vi "BuildCustomDashBoardData.vi"() -> ()   [LabVIEW 2013]
doc: "This VI builds data and sends it back to the dashboard PC program. By default it sends back the raw values for the first analog, digital, and solenoid module. Modify it to send back the data you want to view. Consider adding higher level data to the Dashboard Datatype.ctl and to this VI. Then update the Dashboard to display the data however you like.\n\nThis software is licensed. Open the labview\\readme\\WPI Robotics Library Open Source License.txt file for more information."
uses:
  typedefs/Dashboard/DashboardEnable.ctl
  typedefs/fg_typedef.ctl
  <vilib>/Rock Robotics/SystemInterfaces/Typedef/FPGA_TypedefDigitalModule.ctl
  typedefs/Dashboard/dash dio.ctl
  typedefs/Dashboard/misc dash data.ctl
  typedefs/Dashboard/dashboard safety status data.ctl
  typedefs/Dashboard/dash error type def.ctl
  <vilib>/Rock Robotics/SystemInterfaces/System/FPGA_SystemGet.vi
  <vilib>/NI_Real-Time Target Support.lvlib
  <vilib>/Rock Robotics/WPI/DriverStation/WPI_DriverStationDigitalData.ctl
  typedefs/State Machine/subStates.ctl
  typedefs/Dashboard/custom dash data.ctl
  typedefs/Dashboard/Dashboard Datatype.ctl
panel:
  out "Errors":errorcluster
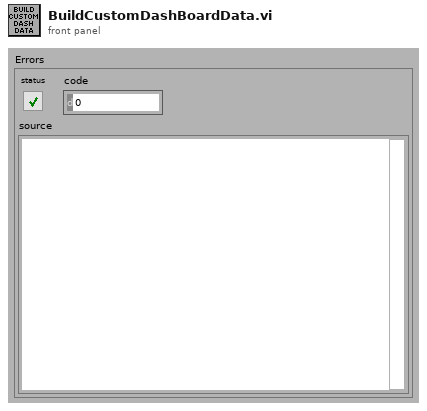
[diagram p1: front panel]
types:
  T1 = typedef "Dashboard Datatype.ctl" = cluster{cluster{"AnalogModule[0]":cluster{"Channel[0]":sgl, "Channel[1]":sgl, "Channel[2]":sgl, "Channel[3]":sgl, "Channel[4]":sgl, "Channel[5]":sgl, "Channel[6]":sgl, "Channel[7]":sgl}, "AnalogModule[1]":cluster{"Channel[0]":sgl, "Channel[1]":sgl, "Channel[2]":sgl, "Channel[3]":sgl, "Channel[4]":sgl, "Channel[5]":sgl, "Channel[6]":sgl, "Channel[7]":sgl}}, cluster{"DigitalModule[0]":T2, "DigitalModule[1]":T2}, "Solenoid":u8}
  T2 = typedef "WPI_DriverStationDigitalData.ctl" = cluster{"Relay Fwd":u8, "Relay Rev":u8, "GPIO":u16, "GPIO_OE":u16, "PWM":cluster{"PWM[0]":u8, "PWM[1]":u8, "PWM[2]":u8, "PWM[3]":u8, "PWM[4]":u8, "PWM[5]":u8, "PWM[6]":u8, "PWM[7]":u8, "PWM[8]":u8, "PWM[9]":u8}}
  T3 = typedef "custom dash data.ctl" = cluster{"Motors":cluster{"Pickup Motor":dbl, "Pickup Belt":dbl, "Pickup Distance ":dbl, "Pickup Rate":dbl, "Right Motor Rate":dbl, "Left Motor Rate":dbl, "Right Motor Distance":dbl, "Left Motor Distance":dbl}, "substates":cluster{"Latch":T4, "Pickup Arm":T4, "Belts":T4, "Shooter":T4, "Drive":T4}, "Safeties":cluster{"Arm Safety":bool, "Arm Limit":bool}, "Performance":cluster{"CPU Usage":dbl, "Vision mSPI":u32, "Main mSPI":u32}, "Vision Enabled?":bool, "Can Shoot Safely?":bool, "Timeout Error":cluster{"# of Timeouts":u32, "Time Out Error This Match":bool}, "Error FG Data":cluster{"Errors Present":bool, "Errors":string}, "Vision Data":cluster{"Hot Goal Present?":bool, "distance":dbl}}
  T4 = typedef "subStates.ctl" = enum16{"null", "wait", "driver control", "auto", "manual override", "hold position", "rotate", "pickup", "pass", "recover pass", "load", "goto shoot", "shoot high goal", "shoot low goal", "cancel arm", "cancel shooter", "end", "test"}
  T5 = typedef "fg_typedef.ctl" = enum16{"Get", "Set"}
  T6 = cluster{"# of Timeouts":u32, "Time Out Error This Match":bool}
  T7 = typedef "FPGA_TypedefDigitalModule.ctl" = enum16{"Digital Module 1", "Digital Module 2"}
  T8 = typedef "dash dio.ctl" = cluster{"Relay Forward":u8, "Relay Reverse":u8, u32, u32, cluster{"[0]":u8, "[1]":u8, "[2]":u8, "[3]":u8, "[4]":u8, "[5]":u8, "[6]":u8, "[7]":u8, "[8]":u8, "[9]":u8}}[]
  T9 = typedef "misc dash data.ctl" = cluster{"Total (%)":dbl, "Vision mSPI":u32, "Main mSPI":u32, "Vision":cluster{"Hot Goal Present?":bool, "distance":dbl}, "Enabled?":bool, "Safety Data":T10}
  T10 = typedef "dashboard safety status data.ctl" = cluster{"At Distance Limit":bool, "No Rate Read":bool, "Encoder Disconnected":bool, "Encoder Directional Issue":bool}
  T11 = typedef "dash error type def.ctl" = cluster{"Timeout Data":cluster{"# of Timeouts":u32, "Time Out Error This Match":bool}, "Can Shoot Safely?":bool}
  T12 = typedef "DashboardEnable.ctl" = cluster{"Analog Module 1":bool[], "Analog Module 2":bool[], "Digital Module 1":bool, "Digital Module 2":bool, "Solenoid Module":bool}
  T13 = cluster{"AnalogModule[0]":cluster{"Channel[0]":sgl, "Channel[1]":sgl, "Channel[2]":sgl, "Channel[3]":sgl, "Channel[4]":sgl, "Channel[5]":sgl, "Channel[6]":sgl, "Channel[7]":sgl}, "AnalogModule[1]":cluster{"Channel[0]":sgl, "Channel[1]":sgl, "Channel[2]":sgl, "Channel[3]":sgl, "Channel[4]":sgl, "Channel[5]":sgl, "Channel[6]":sgl, "Channel[7]":sgl}}
  T14 = cluster{"DigitalModule[0]":T2, "DigitalModule[1]":T2}
  T15 = typedef "vision data.ctl" = cluster{"x":dbl, "y":dbl, "area":dbl, "width":dbl, "height":dbl, "Hot Goal Present?":bool, "distance":dbl}
  T16 = cluster{"Channel[0]":sgl, "Channel[1]":sgl, "Channel[2]":sgl, "Channel[3]":sgl, "Channel[4]":sgl, "Channel[5]":sgl, "Channel[6]":sgl, "Channel[7]":sgl}[]
  T17 = cluster{"Channel[0]":sgl, "Channel[1]":sgl, "Channel[2]":sgl, "Channel[3]":sgl, "Channel[4]":sgl, "Channel[5]":sgl, "Channel[6]":sgl, "Channel[7]":sgl}
  T18 = cluster{"AnalogModule[0][0]":sgl, "AnalogModule[0][1]":sgl, "AnalogModule[0][2]":sgl, "AnalogModule[0][3]":sgl, "AnalogModule[0][4]":sgl, "AnalogModule[0][5]":sgl, "AnalogModule[0][6]":sgl, "AnalogModule[0][7]":sgl}
  T19 = cluster{"[0]":cluster{"Channel[0]":sgl, "Channel[1]":sgl, "Channel[2]":sgl, "Channel[3]":sgl, "Channel[4]":sgl, "Channel[5]":sgl, "Channel[6]":sgl, "Channel[7]":sgl}, "[1]":cluster{"Channel[0]":sgl, "Channel[1]":sgl, "Channel[2]":sgl, "Channel[3]":sgl, "Channel[4]":sgl, "Channel[5]":sgl, "Channel[6]":sgl, "Channel[7]":sgl}}
  T20 = typedef "FPGA_DIODevRef.ctl" = cluster{"DevStatus":errorcluster, "Module":T7}
  T21 = cluster{"[0]":u8, "[1]":u8, "[2]":u8, "[3]":u8, "[4]":u8, "[5]":u8, "[6]":u8, "[7]":u8, "[8]":u8, "[9]":u8}
  T22 = typedef "FPGA_SolenoidDevRef.ctl" = cluster{"DevStatus":errorcluster, "Module":T23}
  T23 = typedef "FPGA_TypedefSolenoidModule.ctl" = enum16{"Solenoid Module 1", "Solenoid Module 2"}
  T24 = cluster{"Pickup Motor":dbl, "Pickup Belt":dbl, "Pickup Distance ":dbl, "Pickup Rate":dbl, "Right Motor Rate":dbl, "Left Motor Rate":dbl, "Right Motor Distance":dbl, "Left Motor Distance":dbl}
  T25 = cluster{"CPU Usage":dbl, "Vision mSPI":u32, "Main mSPI":u32}
  T26 = cluster{"Hot Goal Present?":bool, "distance":dbl}
  T27 = typedef "WPI_EncoderDevRef.ctl" = cluster{"DevStatus":errorcluster, "EncoderIndex":T28, "CounterIndex":T29, "DistancePerCount":dbl, "Decoding Type":T30}
  T28 = typedef "FPGA_EncoderIdx.ctl" = enum8{"Enc 0", "Enc 1", "Enc 2", "Enc 3", "Invalid"}
  T29 = typedef "FPGA_CounterCtrSystemIndex.ctl" = enum8{"Ctr 0", "Ctr 1", "Ctr 2", "Ctr 3", "Ctr 4", "Ctr 5", "Ctr 6", "Ctr 7", "Invalid"}
  T30 = typedef "WPI_EncoderType.ctl" = enum16{"1x", "2x", "4x"}
  T31 = typedef "WPI_MotorControlDeviceRef.ctl" = cluster{"DeviceStatus":errorcluster, "Type":enum16{"PWM", "CAN"}, "PWM":cluster{"Digital Module":T7, "PWM Channel":T32, "DeadBand":T33}, "CAN":cluster{"Device Number":u8, "Control Mode":T34, "Semaphore":T35, "Max Vout":dbl}, "Invert":bool, "TransformRef":T36, "InvTransformRef":T36}
  T32 = typedef "FPGA_DIOPWMChannel.ctl" = enum8{"PWM 1", "PWM 2", "PWM 3", "PWM 4", "PWM 5", "PWM 6", "PWM 7", "PWM 8", "PWM 9", "PWM 10", "Invalid"}
  T33 = typedef "WPI_PWMDeadband.ctl" = cluster{"Name":string, "maxPositivePwm":i32, "minPositivePwm":i32, "centerPwm":i32, "maxNegativePwm":i32, "minNegativePwm":i32, "angularRange":u16}
  T34 = typedef "WPI_CANJaguar_ControlMode.ctl" = enum8{"Percent VBus", "Current", "Speed", "Position", "Voltage"}
  T35 = typedef "Semaphore RefNum" = refnum<k1>
  T36 = typedef "WPI_PWMTransform_ConPane.ctl" = refnum<vi>
  T37 = typedef "NI_Real-Time Target Support.lvlib/RT CPU Load.ctl" = cluster{"Total (%)":dbl, "Time Critical (%)":dbl, "Timed Structures (%)":dbl, "High (%)":dbl, "Above Normal (%)":dbl, "Normal (%)":dbl, "Background (%)":dbl, "Idle (%)":dbl, "ISR (%)":dbl}
  T38 = cluster{"Vision mSPI":u32, "Main mSPI":u32, "Dash mSPI":u32}
  T39 = cluster{"Relay Forward":u8, "Relay Reverse":u8, u32, u32, cluster{"[0]":u8, "[1]":u8, "[2]":u8, "[3]":u8, "[4]":u8, "[5]":u8, "[6]":u8, "[7]":u8, "[8]":u8, "[9]":u8}}
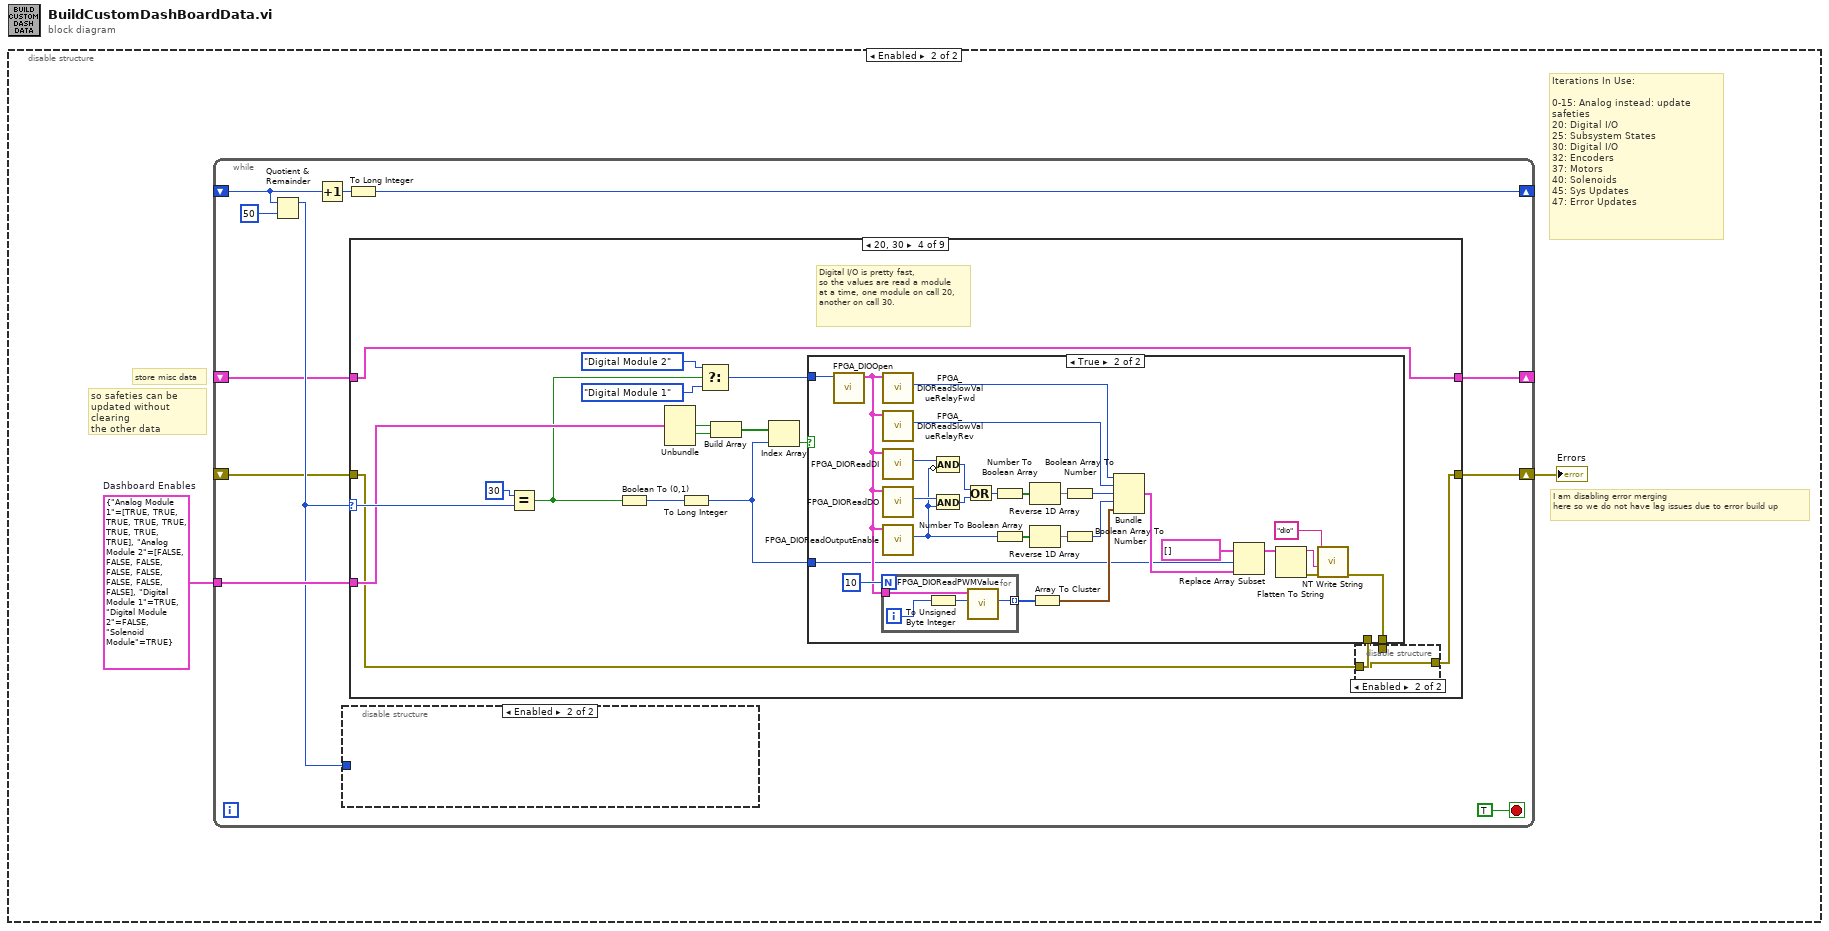
[diagram p0: block diagram]
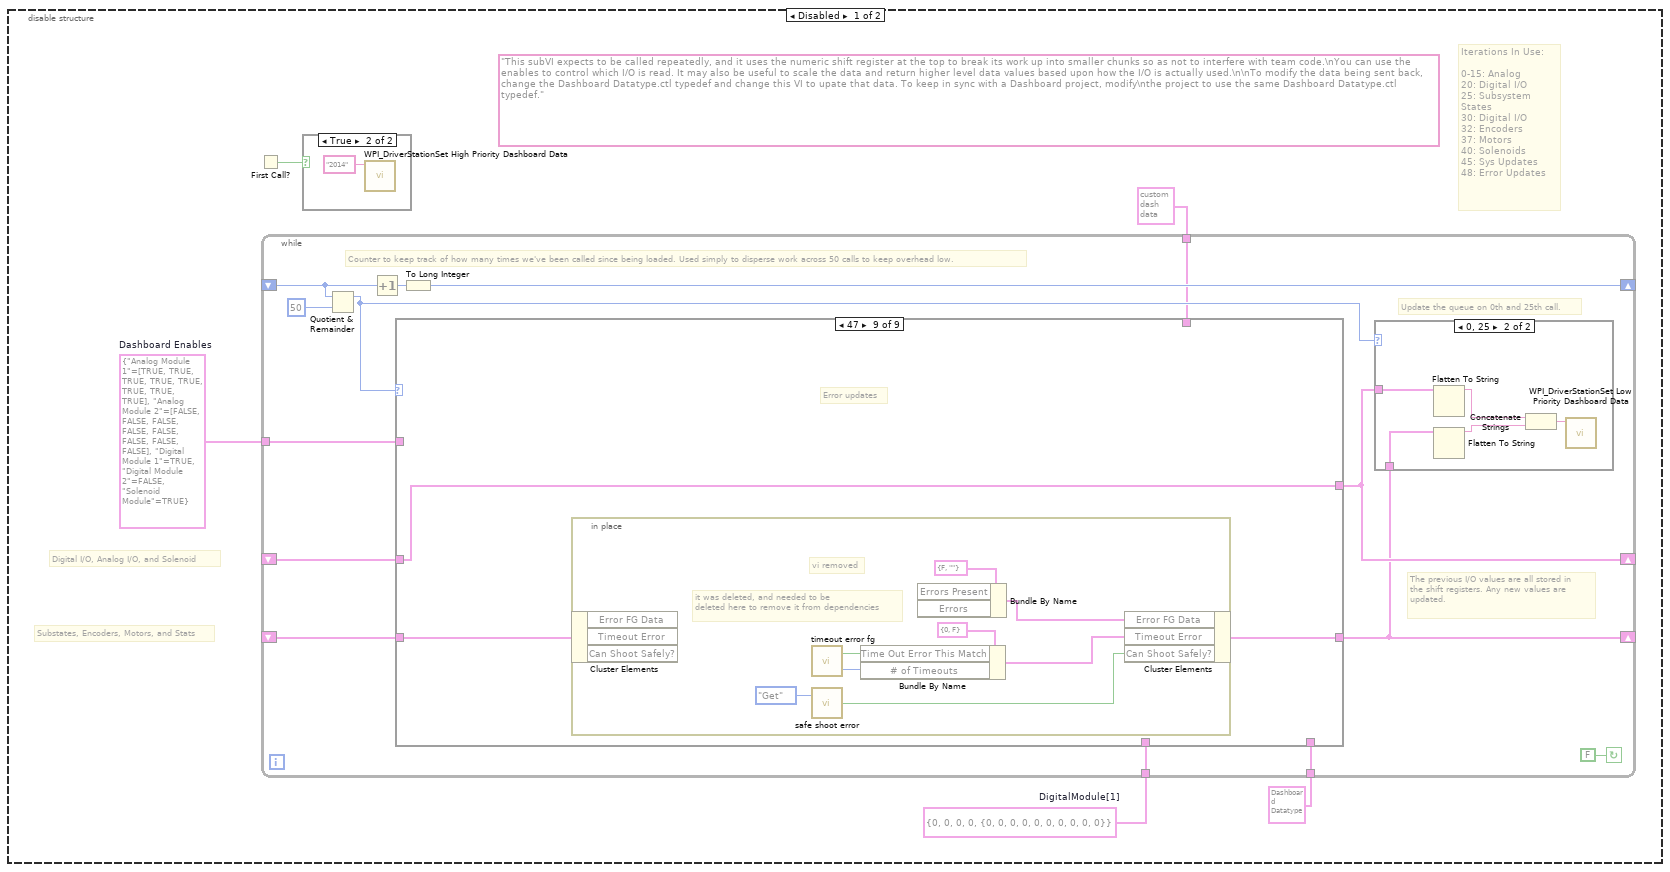
[diagram p2: hidden frame]
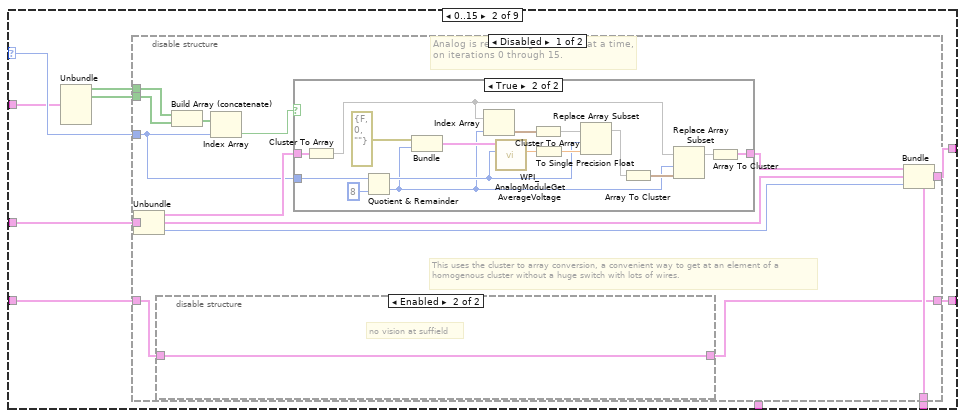
[diagram p6: hidden frame]
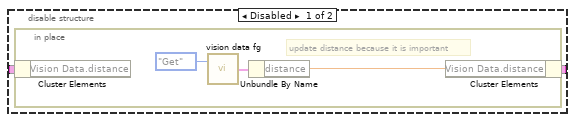
[diagram p8: hidden frame]
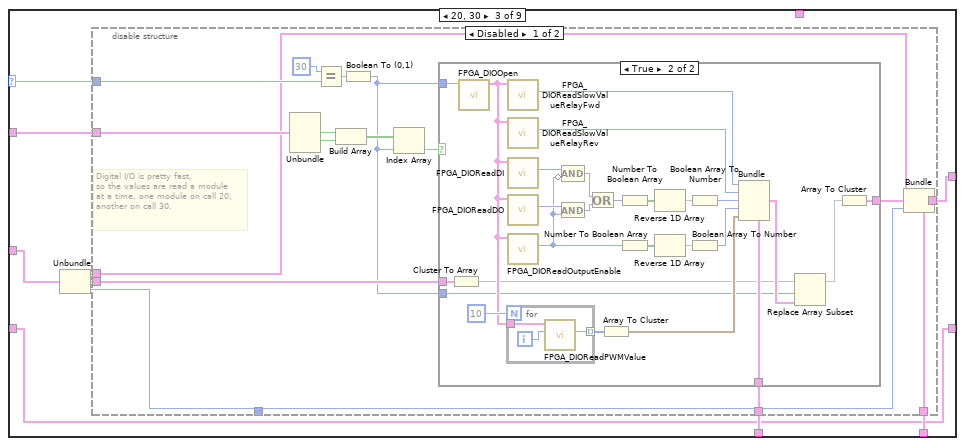
[diagram p10: hidden frame]
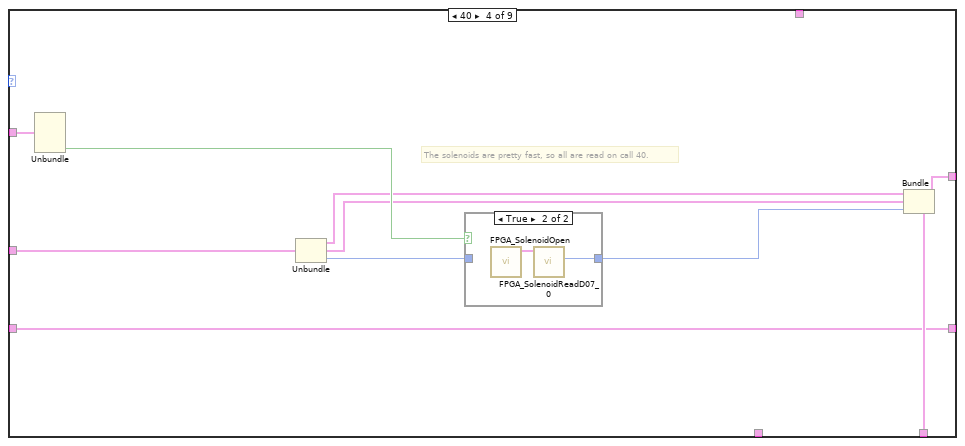
[diagram p13: hidden frame]
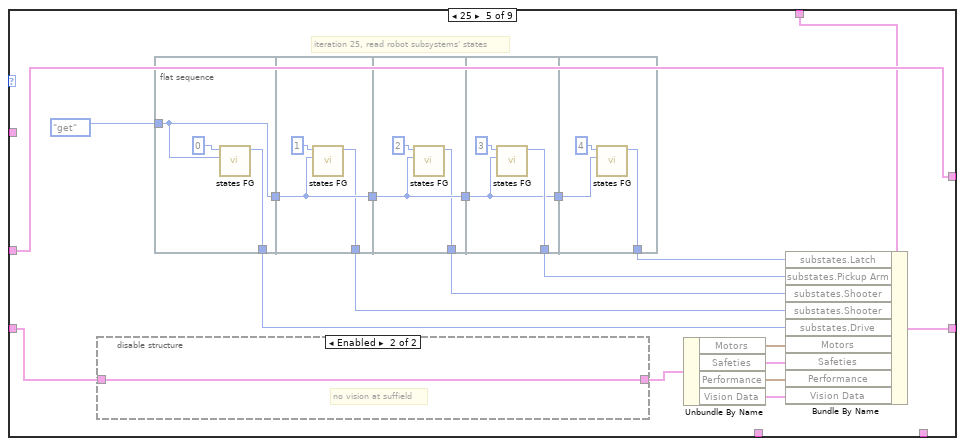
[diagram p15: hidden frame]
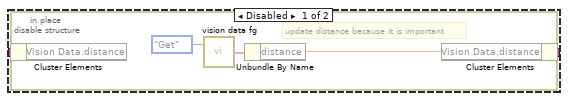
[diagram p16: hidden frame]
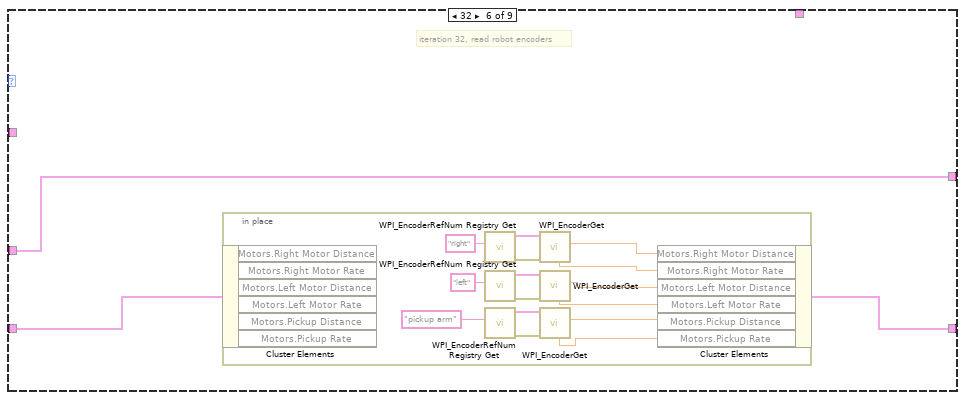
[diagram p17: hidden frame]
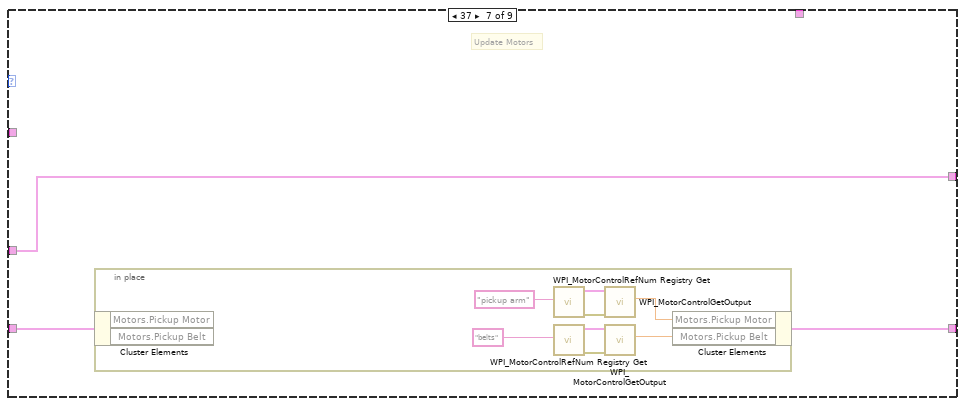
[diagram p18: hidden frame]
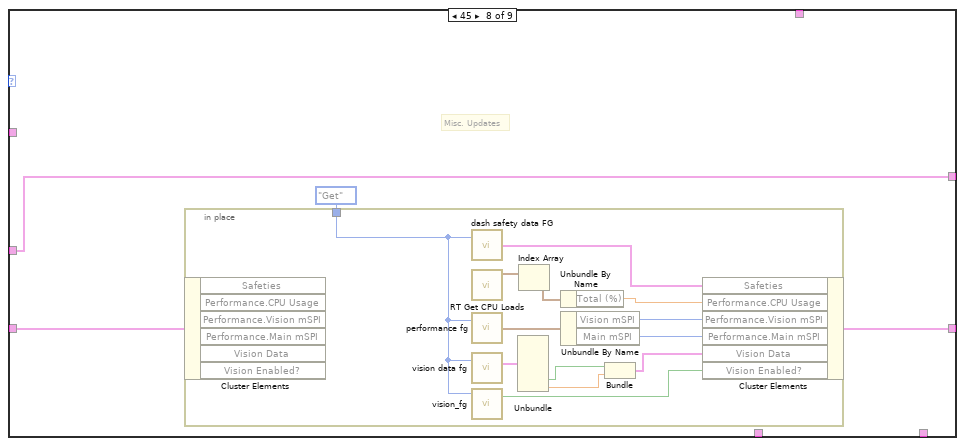
[diagram p19: hidden frame]
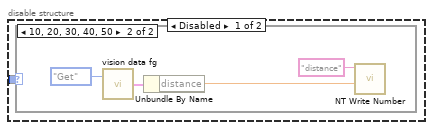
[diagram p20: hidden frame]
diagram:
  n1 = disable-structure shown="Enabled" {
    frame Disabled {
      w1 = T12 {"Analog Module 1"=[TRUE, TRUE, TRUE, TRUE, TRUE, TRUE, TRUE, TRUE], "Analog Module 2"=[FALSE, FALSE, FALSE, FALSE, FALSE, FALSE, FALSE, FALSE], "Digital Module 1"=TRUE, "Digital Module 2"=FALSE, "Solenoid Module"=TRUE}  # Dashboard Enables
      w2 = T2 {"Relay Fwd"=0, "Relay Rev"=0, "GPIO"=0, "GPIO_OE"=0, "PWM"={"PWM[0]"=0, "PWM[1]"=0, "PWM[2]"=0, "PWM[3]"=0, "PWM[4]"=0, "PWM[5]"=0, "PWM[6]"=0, "PWM[7]"=0, "PWM[8]"=0, "PWM[9]"=0}}  # DigitalModule[1]
      (unwired) "This subVI expects to be called repeatedly, and it uses the numeric shift register at the top to break its work up into smaller chunks so as not to interfere with team code.\nYou can use the enables to control which I/O is read. It may also be useful to scale the data and return higher level data values based upon how the I/O is actually used.\n\nTo modify the data being sent back, change the Dashboard Datatype.ctl typedef and change this VI to upate that data. To keep in sync with a Dashboard project, modify\nthe project to use the same Dashboard Datatype.ctl typedef."
      # "Iterations In Use:\n\n0-15: Analog\n20: Digital I/O \n25: Subsystem States\n30: Digital I/O\n32: Encoders\n37: Motors\n40: Solenoids\n45: Sys Updates\n48: Error Updates"
      # "Substates, Encoders, Motors, and Stats"
      # "Digital I/O, Analog I/O, and Solenoid"
      n2 = First Call?() -> (First Call?: T/F=w3:bool)
      n3 = while {
        shift-right: [w13] -> _
        shift-left: _ -> [w15]
        shift-right: [w10] -> _
        shift-left: _ -> [w18]
        tunnel: w2 -> [w17]
        tunnel: T1 {{"AnalogModule[0]"={"Channel[0]"=0.0, "Channel[1]"=0.0, "Channel[2]"=0.0, "Channel[3]"=0.0, "Channel[4]"=0.0, "Channel[5]"=0.0, "Channel[6]"=0.0, "Channel[7]"=0.0}, "AnalogModule[1]"={"Channel[0]"=0.0, "Channel[1]"=0.0, "Channel[2]"=0.0, "Channel[3]"=0.0, "Channel[4]"=0.0, "Channel[5]"=0.0, "Channel[6]"=0.0, "Channel[7]"=0.0}}, {"DigitalModule[0]"={"Relay Fwd"=0, "Relay Rev"=0, "GPIO"=0, "GPIO_OE"=0, "PWM"={"PWM[0]"=0, "PWM[1]"=0, "PWM[2]"=0, "PWM[3]"=0, "PWM[4]"=0, "PWM[5]"=0, "PWM[6]"=0, "PWM[7]"=0, "PWM[8]"=0, "PWM[9]"=0}}, "DigitalModule[1]"={"Relay Fwd"=0, "Relay Rev"=0, "GPIO"=0, "GPIO_OE"=0, "PWM"={"PWM[0]"=0, "PWM[1]"=0, "PWM[2]"=0, "PWM[3]"=0, "PWM[4]"=0, "PWM[5]"=0, "PWM[6]"=0, "PWM[7]"=0, "PWM[8]"=0, "PWM[9]"=0}}}, "Solenoid"=0} ("Dashboard Data") -> [w12]
        tunnel: w1 -> [w11]
        shift-right: [w7] -> _
        shift-left: _ -> [w8]
        tunnel: T3 {"Motors"={"Pickup Motor"=0.0, "Pickup Belt"=0.0, "Pickup Distance "=0.0, "Pickup Rate"=0.0, "Right Motor Rate"=0.0, "Left Motor Rate"=0.0, "Right Motor Distance"=0.0, "Left Motor Distance"=0.0}, "substates"={"Latch"=enum."null", "Pickup Arm"=enum."null", "Belts"=enum."null", "Shooter"=enum."null", "Drive"=enum."null"}, "Safeties"={"Arm Safety"=FALSE, "Arm Limit"=FALSE}, "Performance"={"CPU Usage"=0.0, "Vision mSPI"=0, "Main mSPI"=0}, "Vision Enabled?"=FALSE, "Can Shoot Safely?"=FALSE, "Timeout Error"={"# of Timeouts"=0, "Time Out Error This Match"=FALSE}, "Error FG Data"={"Errors Present"=FALSE, "Errors"=""}, "Vision Data"={"Hot Goal Present?"=FALSE, "distance"=0.0}} ("Custom Dash Data") -> [w9]
        stop <- FALSE continue-if-true
        # "Counter to keep track of how many times we've been called since being loaded. Used simply to disperse work across 50 calls to keep overhead low."
        # "Update the queue on 0th and 25th call."
        # "The previous I/O values are all stored in\nthe shift registers. Any new values are\nupdated."
        n4 = Quotient & Remainder(x=w15, y=50) -> (x-y*floor(x/y)=w14:i32)  [unwired: 1 out]
        n5 = Increment(x=w15) -> (x+1=w20:i32)
        n6 = case shown="47" w14 {
          selector: w14 -> [_ w35 w82 _ _ _ _ _ _]
          tunnel: [w27 w31 w77 w136 w151 w184 w203 w214 w230] -> w10
          tunnel: w18 -> [w27 w30 w79 w138 w151 w184 w203 w214 w230]
          tunnel: w17 -> [_ _ w83 _ _ _ _ _ _]
          tunnel: w12 -> [_ w36 w78 w135 _ _ _ _ _]
          tunnel: w11 -> [_ w34 w81 w139 _ _ _ _ _]
          tunnel: w9 -> [_ _ _ _ w149 _ _ _ _]
          tunnel: [w26 w28 w76 w132 w150 w185 w202 w215 w231] -> w7
          tunnel: w8 -> [w26 w29 w76 w132 w145 w183 w201 w213 w229]
          frame Default {
            # "Don't update any I/O"
          }
          frame 0..15 {
            n7 = Unbundle(w34) -> ("Analog Module 1"=w33:bool[], "Analog Module 2"=w32:bool[])  [unwired: 3 out]
            n8 = disable-structure shown="Disabled" {
              disable-tunnel: w36 -> [w47 _]
              disable-tunnel: w35 -> [w45 _]
              disable-tunnel: w33 -> [w44 _]
              disable-tunnel: w32 -> [w43 _]
              disable-tunnel: [w42 _] -> w31
              disable-tunnel: w30 -> [w41 _]
              disable-tunnel: w29 -> [w38 _]
              disable-tunnel: [w37 _] -> w28
              frame Disabled {
                # "This uses the cluster to array conversion, a convenient way to get at an element of a\nhomogenous cluster without a huge switch with lots of wires."
                # "Analog is read a single channel at a time,\non iterations 0 through 15."
                n9 = Unbundle(w41) -> (w46:T13, w40:T14, "Solenoid"=w39:u8)
                n10 = disable-structure shown="Enabled" {
                  disable-tunnel: w38 -> [w69 w73]
                  disable-tunnel: [w68 w73] -> w37
                  frame Disabled {
                    n11 = in-place {
                      # "update distance because it is important"
                      n12 = in-place-cluster #1(w69) -> ()  [unwired: 1 out]
                      n13 = call "vision data fg.vi"("Menu"=fg_typedef."Get") -> ("Output"=w71:T15)  [unwired: 1 in]
                      n14 = Unbundle By Name(w71) -> ("distance"=w70:dbl)
                      n15 = in-place-cluster #1("Vision Data.distance"=w70) -> (w68:T3)
                    }
                  }
                  frame Enabled {
                    # "no vision at suffield"
                  }
                }
                n16 = Build Array (concatenate)(w44, w43) -> (w49:bool[])
                n17 = Index Array(array=w49, index=w45) -> (element=w50:bool)
                n18 = case shown="True" w50 {
                  tunnel: w45 -> [_ w58]
                  tunnel: [w51 w55] -> w48
                  tunnel: w46 -> [w51 w54]
                  frame False {
                  }
                  frame True {
                    n19 = Cluster To Array(cluster=w54) -> (array=w53:T16)
                    n20 = Quotient & Remainder(x=w58, y=8) -> (x-y*floor(x/y)=w57:i32, floor(x/y)=w52:i32)
                    n21 = Bundle("DevStatus"=errorcluster {"status"=FALSE, "code"=0, "source"=""}, w52) -> (w66:cluster{"DevStatus":errorcluster, i32})  [unwired: 1 out]
                    n22 = Index Array(array=w53, index=w52) -> (element=w60:T17)
                    n23 = call <vilib>:"WPI_AnalogModuleGetAverageVoltage.vi"("Channel"=w57, "AnalogModuleDevStatus"=w66) -> ("Average Voltage"=w63:dbl)  [unwired: 1 in, 8 out]
                    n24 = Cluster To Array(cluster=w60) -> (array=w59:sgl[])
                    n25 = To Single Precision Float(number=w63) -> (single precision float=w62:sgl)
                    n26 = Replace Array Subset(array=w59, new element=w62, index=w57) -> (w61:sgl[])
                    n27 = Array To Cluster(array=w61) -> (cluster=w65:T18)
                    n28 = Replace Array Subset(array=w53, new element=w65, index=w52) -> (w56:T16)
                    n29 = Array To Cluster(array=w56) -> (cluster=w55:T19)
                  }
                }
                n30 = Bundle(cluster=w47, w48, w40, "Solenoid"=w39) -> (w42:T1)
              }
              frame Enabled {
              }
            }
          }
          frame 20, 30 {
            n31 = Unbundle(w79) -> (w75:T13, w80:T14, "Solenoid"=w74:u8)
            n32 = disable-structure shown="Disabled" {
              disable-tunnel: w83 -> [w99 _]
              disable-tunnel: w82 -> [w95 _]
              disable-tunnel: w81 -> [w93 _]
              disable-tunnel: w80 -> [w90 _]
              disable-tunnel: w78 -> [w88 _]
              disable-tunnel: [w87 _] -> w77
              disable-tunnel: w75 -> [w85 _]
              disable-tunnel: w74 -> [w84 _]
              frame Disabled {
                # "Digital I/O is pretty fast,\nso the values are read a module\nat a time, one module on call 20,\nanother on call 30."
                n33 = Unbundle(w93) -> ("Digital Module 1"=w92:bool, "Digital Module 2"=w91:bool)  [unwired: 3 out]
                n34 = Equal?(x=30, y=w95) -> (x = y?=w97:bool)
                n35 = Build Array(w92, w91) -> (w94:bool[])
                n36 = Boolean To (0,1)(Boolean=w97) -> (0, 1=w86:i16)
                n37 = Index Array(array=w94, index=w86) -> (element=w96:bool)
                n38 = case shown="True" w96 {
                  tunnel: w99 -> [_ w108]
                  tunnel: [w100 w101] -> w89
                  tunnel: w86 -> [_ w106]
                  tunnel: w86 -> [_ w105]
                  tunnel: w90 -> [w100 w104]
                  frame False {
                  }
                  frame True {
                    n39 = Cluster To Array(cluster=w104) -> (array=w103:T2[])
                    n40 = call <vilib>:"FPGA_DIOOpen.vi"("Module (Module 1)"=w106) -> ("DIODeviceRef"=w124:T20)  [unwired: 1 in, 9 out]
                    n41 = for {
                      N: 10 -> [_]
                      tunnel: w124 -> [w129]
                      tunnel: [w127] -> w125 mode=indexing
                      i -> [w128]
                      n42 = call <vilib>:"FPGA_DIOReadPWMValue.vi"("PWMChannel"=w128, "DIODeviceRef In"=w129) -> ("PWMValue"=w127:u8)  [unwired: 1 in, 8 out]
                    }
                    n43 = call <vilib>:"FPGA_DIOReadSlowValueRelayFwd.vi"("DIODeviceRef In"=w124) -> ("Relay Forward"=w117:u8)  [unwired: 1 in, 9 out]
                    n44 = call <vilib>:"FPGA_DIOReadSlowValueRelayRev.vi"("DIODeviceRef In"=w124) -> ("Relay Reverse"=w118:u8)  [unwired: 1 in, 9 out]
                    n45 = call <vilib>:"FPGA_DIOReadDI.vi"("DIODeviceRef In"=w124) -> ("DI"=w122:u16)  [unwired: 1 in, 9 out]
                    n46 = call <vilib>:"FPGA_DIOReadDO.vi"("DIODeviceRef In"=w124) -> ("DO"=w121:u16)  [unwired: 1 in, 9 out]
                    n47 = call <vilib>:"FPGA_DIOReadOutputEnable.vi"("DIODeviceRef In"=w124) -> ("OutputEnable"=w112:u16)  [unwired: 1 in, 9 out]
                    n48 = And(x=w121, y=w112) -> (x .and. y?=w120:u16)
                    n49 = Compound Arithmetic op=AND(w122, invert w112) -> (w119:u16)
                    n50 = Or(x=w119, y=w120) -> (x .or. y?=w110:u16)
                    n51 = Array To Cluster(array=w125) -> (cluster=w123:T21)
                    n52 = Number To Boolean Array(number=w110) -> (Boolean array=w115:bool[])
                    n53 = Number To Boolean Array(number=w112) -> (Boolean array=w114:bool[])
                    n54 = Reverse 1D Array(array=w115) -> (reversed array=w116:bool[])
                    n55 = Reverse 1D Array(array=w114) -> (reversed array=w113:bool[])
                    n56 = Boolean Array To Number(Boolean array=w116) -> (number=w109:u32)
                    n57 = Boolean Array To Number(Boolean array=w113) -> (number=w111:u32)
                    n58 = Bundle(cluster=w108, "Relay Fwd"=w117, "Relay Rev"=w118, "GPIO"=w109, "GPIO_OE"=w111, "PWM"=w123) -> (w107:T2)
                    n59 = Replace Array Subset(array=w103, new element=w107, index=w105) -> (w102:T2[])
                    n60 = Array To Cluster(array=w102) -> (cluster=w101:cluster{"[0]":T2, "[1]":T2})
                  }
                }
                n61 = Bundle(cluster=w88, w85, w89, "Solenoid"=w84) -> (w87:T1)
              }
              frame Enabled {
              }
            }
          }
          frame 40 {
            # "The solenoids are pretty fast, so all are read on call 40."
            n62 = Unbundle(w139) -> ("Solenoid Module"=w133:bool)  [unwired: 4 out]
            n63 = Unbundle(w138) -> (w131:T13, w130:T14, "Solenoid"=w137:u8)
            n64 = case shown="True" w133 {
              tunnel: [w140 w141] -> w134
              tunnel: w137 -> [w140 _]
              frame False {
              }
              frame True {
                n65 = call <vilib>:"FPGA_SolenoidOpen.vi"() -> ("SolenoidDevRef"=w142:T22)  [unwired: 2 in, 9 out]
                n66 = call <vilib>:"FPGA_SolenoidReadD07_0.vi"("SolenoidDevRef"=w142) -> ("DO7:0"=w141:u8)  [unwired: 1 in, 9 out]
              }
            }
            n67 = Bundle(cluster=w135, w131, w130, "Solenoid"=w134) -> (w136:T1)
          }
          frame 25 {
            # "iteration 25, read robot subsystems' states"
            n68 = disable-structure shown="Enabled" {
              disable-tunnel: w145 -> [w163 w167]
              disable-tunnel: [w162 w167] -> w144
              frame Disabled {
                n69 = in-place {
                  # "update distance because it is important"
                  n70 = in-place-cluster #2(w163) -> ()  [unwired: 1 out]
                  n71 = call "vision data fg.vi"("Menu"=fg_typedef."Get") -> ("Output"=w165:T15)  [unwired: 1 in]
                  n72 = Unbundle By Name(w165) -> ("distance"=w164:dbl)
                  n73 = in-place-cluster #2("Vision Data.distance"=w164) -> (w162:T3)
                }
              }
              frame Enabled {
                # "no vision at suffield"
              }
            }
            n74 = flat-sequence {
              tunnel: enum16{"set", "get"}."get" ("menu (get)") -> [w170]
              tunnel: [w170] -> w158
              tunnel: [w168] -> w152
              tunnel: [w173] -> w159
              tunnel: w158 -> [w173]
              tunnel: [w171] -> w153
              tunnel: [w176] -> w160
              tunnel: w159 -> [w176]
              tunnel: [w174] -> w154
              tunnel: w160 -> [w177]
              tunnel: [w178] -> w155
              tunnel: [w177] -> w157
              tunnel: w157 -> [w181]
              tunnel: [w180] -> w156
              frame #0 {
                n75 = call "states FG.vi"("menu (get)"=w170, "Loop ID"=0) -> ("subState out"=w168:T4)  [unwired: 6 in, 3 out]
              }
              frame #1 {
                n76 = call "states FG.vi"("menu (get)"=w173, "Loop ID"=1) -> ("subState out"=w171:T4)  [unwired: 6 in, 3 out]
              }
              frame #2 {
                n77 = call "states FG.vi"("menu (get)"=w176, "Loop ID"=2) -> ("subState out"=w174:T4)  [unwired: 6 in, 3 out]
              }
              frame #3 {
                n78 = call "states FG.vi"("menu (get)"=w177, "Loop ID"=3) -> ("subState out"=w178:T4)  [unwired: 6 in, 3 out]
              }
              frame #4 {
                n79 = call "states FG.vi"("menu (get)"=w181, "Loop ID"=4) -> ("subState out"=w180:T4)  [unwired: 6 in, 3 out]
              }
            }
            n80 = Unbundle By Name(w144) -> ("Motors"=w143:T24, "Safeties"=w148:cluster{"Arm Safety":bool, "Arm Limit":bool}, "Performance"=w147:T25, "Vision Data"=w146:T26)
            n81 = Bundle By Name(cluster=w149, "substates.Latch"=w156, "substates.Pickup Arm"=w155, "substates.Shooter"=w154, "substates.Shooter"=w153, "substates.Drive"=w152, "Motors"=w143, "Safeties"=w148, "Performance"=w147, "Vision Data"=w146) -> (w150:T3)
          }
          frame 32 {
            # "iteration 32, read robot encoders"
            n82 = in-place {
              n83 = in-place-cluster #3(w183) -> ()  [unwired: 6 out]
              n84 = call <vilib>:"WPI_EncoderRefNum Registry Get.vi"("refnum name"="right") -> ("error out"=w192:errorcluster, "EncoderDevRef"=w193:T27)  [unwired: 9 in]
              n85 = call <vilib>:"WPI_EncoderRefNum Registry Get.vi"("refnum name"="left") -> ("error out"=w195:errorcluster, "EncoderDevRef"=w194:T27)  [unwired: 9 in]
              n86 = call <vilib>:"WPI_EncoderRefNum Registry Get.vi"("refnum name"="pickup arm") -> ("error out"=w199:errorcluster, "EncoderDevRef"=w200:T27)  [unwired: 9 in]
              n87 = call <vilib>:"WPI_EncoderGet.vi"("error in (no error)"=w192, "EncoderDevRef"=w193) -> ("Distance"=w187:dbl, "Rate"=w186:dbl)  [unwired: 4 in, 4 out]
              n88 = call <vilib>:"WPI_EncoderGet.vi"("error in (no error)"=w195, "EncoderDevRef"=w194) -> ("Distance"=w188:dbl, "Rate"=w189:dbl)  [unwired: 4 in, 4 out]
              n89 = call <vilib>:"WPI_EncoderGet.vi"("error in (no error)"=w199, "EncoderDevRef"=w200) -> ("Distance"=w197:dbl, "Rate"=w196:dbl)  [unwired: 4 in, 4 out]
              n90 = in-place-cluster #3("Motors.Right Motor Distance"=w187, "Motors.Right Motor Rate"=w186, "Motors.Left Motor Distance"=w188, "Motors.Left Motor Rate"=w189, "Motors.Pickup Distance"=w197, "Motors.Pickup Rate"=w196) -> (w185:T3)
            }
          }
          frame 37 {
            # "Update Motors"
            n91 = in-place {
              n92 = in-place-cluster #4(w201) -> ()  [unwired: 2 out]
              n93 = call <vilib>:"WPI_MotorControlRefNum Registry Get.vi"("refnum name"="pickup arm") -> ("error out"=w204:errorcluster, "MotorControlDevRef"=w208:T31)  [unwired: 9 in]
              n94 = call <vilib>:"WPI_MotorControlRefNum Registry Get.vi"("refnum name"="belts") -> ("error out"=w205:errorcluster, "MotorControlDevRef"=w211:T31)  [unwired: 9 in]
              n95 = call <vilib>:"WPI_MotorControlGetOutput.vi"("error in (no error)"=w204, "MotorControlDevRef"=w208) -> ("Output"=w207:dbl)  [unwired: 7 in, 2 out]
              n96 = call <vilib>:"WPI_MotorControlGetOutput.vi"("error in (no error)"=w205, "MotorControlDevRef"=w211) -> ("Output"=w206:dbl)  [unwired: 7 in, 2 out]
              n97 = in-place-cluster #4("Motors.Pickup Motor"=w207, "Motors.Pickup Belt"=w206) -> (w202:T3)
            }
          }
          frame 45 {
            # "Misc. Updates"
            n98 = in-place {
              in-place-border: fg_typedef."Get" ("Menu (Get)") -> [w220]
              n99 = in-place-cluster #5(w213) -> ()  [unwired: 6 out]
              n100 = call "dash safety data FG.vi"("Menu"=w220) -> ("Safety Data Out"=w222:T10)  [unwired: 1 in]
              n101 = call <vilib>:"RT Get CPU Loads.vi"() -> ("CPU loads"=w227:T37[])  [unwired: 10 in, 1 out]
              n102 = call "performance fg.vi"("Menu"=w220) -> ("Output"=w223:T38)  [unwired: 1 in]
              n103 = call "vision data fg.vi"("Menu"=w220) -> ("Output"=w219:T15)  [unwired: 1 in]
              n104 = call "vision_fg.vi"("Menu"=w220) -> ("Enabled?"=w221:bool)  [unwired: 2 in, 1 out]
              n105 = Unbundle(w219) -> ("Hot Goal Present?"=w218:bool, "distance"=w217:dbl)  [unwired: 5 out]
              n106 = Index Array(array=w227) -> (element=w228:T37)  [unwired: 1 in]
              n107 = Unbundle By Name(w228) -> ("Total (%)"=w226:dbl)
              n108 = Unbundle By Name(w223) -> ("Vision mSPI"=w225:u32, "Main mSPI"=w224:u32)
              n109 = Bundle("Hot Goal Present?"=w218, "distance"=w217) -> (w216:T26)  [unwired: 1 in]
              n110 = in-place-cluster #5("Safeties"=w222, "Performance.CPU Usage"=w226, "Performance.Vision mSPI"=w225, "Performance.Main mSPI"=w224, "Vision Data"=w216, "Vision Enabled?"=w221) -> (w215:T3)
            }
          }
          frame 47 {
            # "Error updates"
            n111 = in-place {
              # "it was deleted, and needed to be\ndeleted here to remove it from dependencies"
              # "vi removed"
              n112 = in-place-cluster #6(w229) -> ()  [unwired: 3 out]
              n113 = call "timeout error fg.vi"() -> ("# of Timeouts"=w238:u32, "Time Out Error This Match"=w237:bool)  [unwired: 2 in]
              n114 = call "safe shoot error.vi"("Menu"=fg_typedef."Get") -> ("Can Shoot Safely?"=w234:bool)  [unwired: 1 in]
              n115 = Bundle By Name(cluster=T6 {"# of Timeouts"=0, "Time Out Error This Match"=FALSE}, "Time Out Error This Match"=w237, "# of Timeouts"=w238) -> (w236:T6)
              n116 = Bundle By Name(cluster=cluster{"Errors Present":bool, "Errors":string} {"Errors Present"=FALSE, "Errors"=""}) -> (w232:cluster{"Errors Present":bool, "Errors":string})  [unwired: 2 in]
              n117 = in-place-cluster #6("Error FG Data"=w232, "Timeout Error"=w236, "Can Shoot Safely?"=w234) -> (w231:T3)
            }
          }
        }
        n118 = To Long Integer(number=w20) -> (32bit integer=w13:i32)
        n119 = case shown="0, 25" w14 {
          tunnel: w10 -> [_ w25]
          tunnel: w7 -> [_ w23]
          frame Default {
          }
          frame 0, 25 {
            n120 = Flatten To String(anything=w25) -> (data string=w24:string)  [unwired: 1 in, 4 out]
            n121 = Flatten To String(anything=w23) -> (data string=w21:string)  [unwired: 1 in, 4 out]
            n122 = Concatenate Strings(w24, w21) -> (w22:string)
            n123 = call <vilib>:"WPI_DriverStationSet Low Priority Dashboard Data.vi"("User Data"=w22) -> ()  [unwired: 1 in, 10 out]
          }
        }
      }
      n124 = case shown="True" w3 {
        frame False {
        }
        frame True {
          n125 = call <vilib>:"WPI_DriverStationSet High Priority Dashboard Data.vi"("User Data"="2014") -> ()  [unwired: 10 in, 1 out]
        }
      }
    }
    frame Enabled {
      w241 = T12 {"Analog Module 1"=[TRUE, TRUE, TRUE, TRUE, TRUE, TRUE, TRUE, TRUE], "Analog Module 2"=[FALSE, FALSE, FALSE, FALSE, FALSE, FALSE, FALSE, FALSE], "Digital Module 1"=TRUE, "Digital Module 2"=FALSE, "Solenoid Module"=TRUE}  # Dashboard Enables
      # "I am disabling error merging\nhere so we do not have lag issues due to error build up"
      # "so safeties can be\nupdated without clearing\nthe other data"
      # "store misc data"
      # "Iterations In Use:\n\n0-15: Analog instead: update safeties\n20: Digital I/O \n25: Subsystem States\n30: Digital I/O\n32: Encoders\n37: Motors\n40: Solenoids\n45: Sys Updates\n47: Error Updates"
      n126 = while {
        shift-right: [w249] -> _
        shift-left: _ -> [w250]
        tunnel: w241 -> [w247]
        shift-right: [w245] -> w240
        shift-left: _ -> [w244]
        shift-right: [w243] -> _
        shift-left: _ -> [w242]
        stop <- TRUE stop-if-true
        n127 = Quotient & Remainder(x=w250, y=50) -> (x-y*floor(x/y)=w246:i32)  [unwired: 1 out]
        n128 = Increment(x=w250) -> (x+1=w251:i32)
        n129 = disable-structure shown="Enabled" {
          disable-tunnel: w246 -> [w253 _]
          frame Disabled {
            n130 = case shown="10, 20, 30, 40, 50" w253 {
              frame 0, Default {
              }
              frame 10, 20, 30, 40, 50 {
                n131 = call "vision data fg.vi"("Menu"=fg_typedef."Get") -> ("Output"=w256:T15)  [unwired: 1 in]
                n132 = Unbundle By Name(w256) -> ("distance"=w255:dbl)
                n133 = call <vilib>:"NT Write Number.vi"("Numeric"=w255, "Name"="distance") -> ()  [unwired: 9 in, 1 out]
              }
            }
          }
          frame Enabled {
          }
        }
        n134 = To Long Integer(number=w251) -> (32bit integer=w249:i32)
        n135 = case shown="20, 30" w246 {
          selector: w246 -> [_ w264 _ w336 _ _ _ _ _]
          tunnel: w247 -> [_ w265 _ w335 _ _ w429 _ _]
          tunnel: [w259 w263 w301 w326 w380 w407 w422 w445 w471] -> w245
          tunnel: w244 -> [w259 w262 w300 w327 w379 w406 w418 w444 w469]
          tunnel: [w258 w260 w299 w325 w378 w403 w417 w442 w468] -> w243
          tunnel: w242 -> [w258 w261 w299 w325 w378 w403 w417 _ w468]
          frame Default {
          }
          frame 0..15 {
            # "so update safety data, it is the most important"
            # "we are not using analog"
            n136 = disable-structure shown="Enabled" {
              disable-tunnel: w265 -> [w272 _]
              disable-tunnel: w264 -> [w269 _]
              disable-tunnel: [w267 w296] -> w263
              disable-tunnel: w262 -> [w266 w296]
              disable-tunnel: w261 -> [_ w292]
              disable-tunnel: [_ w291] -> w260
              frame Disabled {
                # "Analog is read a single channel at a time,\non iterations 0 through 15."
                n137 = Unbundle(w272) -> ("Analog Module 1"=w273:bool[], "Analog Module 2"=w274:bool[])  [unwired: 3 out]
                n138 = Build Array (concatenate)(w273, w274) -> (w270:bool[])
                n139 = Index Array(array=w270, index=w269) -> (element=w271:bool)
                n140 = case shown="True" w271 {
                  tunnel: w269 -> [_ w286]
                  tunnel: [w275 w276] -> w268
                  tunnel: w266 -> [w275 _]
                  frame False {
                  }
                  frame True {
                    n141 = Quotient & Remainder(x=w286, y=8) -> (x-y*floor(x/y)=w283:i32, floor(x/y)=w287:i32)
                    n142 = Bundle("DevStatus"=errorcluster {"status"=FALSE, "code"=0, "source"=""}, w287) -> (w289:cluster{"DevStatus":errorcluster, i32})  [unwired: 1 out]
                    n143 = call <vilib>:"NT Read Numeric Array.vi"("Name"="analog") -> ("error out"=w278:errorcluster, "Numeric Array"=w284:dbl[])  [unwired: 9 in]
                    n144 = call <vilib>:"WPI_AnalogModuleGetAverageVoltage.vi"("Channel"=w283, "AnalogModuleDevStatus"=w289) -> ("error out"=w277:errorcluster, "Average Voltage"=w282:dbl)  [unwired: 1 in, 7 out]
                    n145 = Replace Array Subset(array=w284, new element=w282, index=w283) -> (w280:dbl[])
                    n146 = Merge Errors(w278, w277) -> (w279:errorcluster)
                    n147 = call <vilib>:"NT Write Numeric Array.vi"("error in"=w279, "Numeric Array"=w280, "Name"="analog") -> ("error out"=w276:errorcluster)  [unwired: 8 in]
                  }
                }
                n148 = Merge Errors(w268, w266) -> (w267:errorcluster)
              }
              frame Enabled {
                n149 = in-place {
                  n150 = in-place-cluster #7(w292) -> ()  [unwired: 1 out]
                  n151 = call "dash safety data FG.vi"("Menu"=fg_typedef."Get") -> ("Safety Data Out"=w297:T10)  [unwired: 1 in]
                  n152 = in-place-cluster #7("Safety Data"=w297) -> (w291:T9)
                }
                n153 = Flatten To String(anything=w291) -> (data string=w295:string, error out=w293:errorcluster)  [unwired: 1 in, 3 out]
                n154 = call <vilib>:"NT Write String.vi"("error in"=w293, "String"=w295, "Name"="dashdata") -> ()  [unwired: 8 in, 1 out]
              }
            }
          }
          frame 25 {
            w315 = enum16{"set", "get"}."get" ("menu (get)")
            # "update subsystem states"
            n155 = call "states FG.vi"("menu (get)"=w315, "Loop ID"=0) -> ("subState out"=w312:T4)  [unwired: 6 in, 3 out]
            n156 = call "states FG.vi"("menu (get)"=w315, "Loop ID"=1) -> ("subState out"=w313:T4)  [unwired: 6 in, 3 out]
            n157 = call "states FG.vi"("menu (get)"=w315, "Loop ID"=2) -> ("subState out"=w314:T4)  [unwired: 6 in, 3 out]
            n158 = call "states FG.vi"("menu (get)"=w315, "Loop ID"=3) -> ("subState out"=w311:T4)  [unwired: 6 in, 3 out]
            n159 = call "states FG.vi"("menu (get)"=w315, "Loop ID"=4) -> ("subState out"=w310:T4)  [unwired: 6 in, 3 out]
            n160 = To Double Precision Float(number=w312) -> (double precision float=w308:dbl)
            n161 = To Double Precision Float(number=w313) -> (double precision float=w307:dbl)
            n162 = To Double Precision Float(number=w314) -> (double precision float=w306:dbl)
            n163 = To Double Precision Float(number=w311) -> (double precision float=w305:dbl)
            n164 = To Double Precision Float(number=w310) -> (double precision float=w304:dbl)
            n165 = Build Array(w308, w307, w306, w305, w304) -> (w303:dbl[])
            n166 = call <vilib>:"NT Write Numeric Array.vi"("Numeric Array"=w303, "Name"="subsystem_states") -> ("error out"=w302:errorcluster)  [unwired: 9 in]
            n167 = disable-structure shown="Enabled" {
              disable-tunnel: w302 -> [w323 _]
              disable-tunnel: [w322 w324] -> w301
              disable-tunnel: w300 -> [w321 w324]
              frame Disabled {
                n168 = Merge Errors(w323, w321) -> (w322:errorcluster)
              }
              frame Enabled {
              }
            }
          }
          frame 20, 30 {
            # "Digital I/O is pretty fast,\nso the values are read a module\nat a time, one module on call 20,\nanother on call 30."
            n169 = Equal?(x=30, y=w336) -> (x = y?=w333:bool)
            n170 = Boolean To (0,1)(Boolean=w333) -> (0, 1=w334:i16)
            n171 = Unbundle(w335) -> ("Digital Module 1"=w338:bool, "Digital Module 2"=w337:bool)  [unwired: 3 out]
            n172 = To Long Integer(number=w334) -> (32bit integer=w331:i32)
            n173 = Select(t=FPGA_TypedefDigitalModule."Digital Module 2" ("Module (Module 1)"), s=w333, f=FPGA_TypedefDigitalModule."Digital Module 1" ("Module (Module 1)")) -> (s? t:f=w330:T7)
            n174 = Build Array(w338, w337) -> (w339:bool[])
            n175 = Index Array(array=w339, index=w331) -> (element=w340:bool)
            n176 = case shown="True" w340 {
              tunnel: w330 -> [_ w354]
              tunnel: w331 -> [_ w353]
              tunnel: [errorcluster {"status"=FALSE, "code"=0, "source"=""} ("error out") w348] -> w328
              tunnel: w327 -> [_ _]
              frame False {
              }
              frame True {
                n177 = call <vilib>:"FPGA_DIOOpen.vi"("Module (Module 1)"=w354) -> ("DIODeviceRef"=w371:T20)  [unwired: 1 in, 9 out]
                n178 = for {
                  N: 10 -> [_]
                  tunnel: w371 -> [w377]
                  tunnel: [w375] -> w372 mode=indexing
                  i -> [w376]
                  n179 = To Unsigned Byte Integer(number=w376) -> (unsigned 8bit integer=w374:u8)
                  n180 = call <vilib>:"FPGA_DIOReadPWMValue.vi"("PWMChannel"=w374, "DIODeviceRef In"=w377) -> ("PWMValue"=w375:u8)  [unwired: 1 in, 8 out]
                }
                n181 = call <vilib>:"FPGA_DIOReadSlowValueRelayFwd.vi"("DIODeviceRef In"=w371) -> ("Relay Forward"=w364:u8)  [unwired: 1 in, 9 out]
                n182 = call <vilib>:"FPGA_DIOReadSlowValueRelayRev.vi"("DIODeviceRef In"=w371) -> ("Relay Reverse"=w365:u8)  [unwired: 1 in, 9 out]
                n183 = call <vilib>:"FPGA_DIOReadDI.vi"("DIODeviceRef In"=w371) -> ("DI"=w369:u16)  [unwired: 1 in, 9 out]
                n184 = call <vilib>:"FPGA_DIOReadDO.vi"("DIODeviceRef In"=w371) -> ("DO"=w368:u16)  [unwired: 1 in, 9 out]
                n185 = call <vilib>:"FPGA_DIOReadOutputEnable.vi"("DIODeviceRef In"=w371) -> ("OutputEnable"=w359:u16)  [unwired: 1 in, 9 out]
                n186 = And(x=w368, y=w359) -> (x .and. y?=w367:u16)
                n187 = Compound Arithmetic op=AND(w369, invert w359) -> (w366:u16)
                n188 = Or(x=w366, y=w367) -> (x .or. y?=w357:u16)
                n189 = Number To Boolean Array(number=w357) -> (Boolean array=w362:bool[])
                n190 = Number To Boolean Array(number=w359) -> (Boolean array=w361:bool[])
                n191 = Reverse 1D Array(array=w362) -> (reversed array=w363:bool[])
                n192 = Reverse 1D Array(array=w361) -> (reversed array=w360:bool[])
                n193 = Array To Cluster(array=w372) -> (cluster=w370:T21)
                n194 = Boolean Array To Number(Boolean array=w363) -> (number=w356:u32)
                n195 = Boolean Array To Number(Boolean array=w360) -> (number=w358:u32)
                n196 = Bundle("Relay Forward"=w364, "Relay Reverse"=w365, w356, w358, w370) -> (w355:T39)  [unwired: 1 out]
                n197 = Replace Array Subset(array=T8 [], new element=w355, index=w353) -> (w352:T8)
                n198 = Flatten To String(anything=w352) -> (data string=w350:string, error out=w351:errorcluster)  [unwired: 1 in, 3 out]
                n199 = call <vilib>:"NT Write String.vi"("error in"=w351, "String"=w350, "Name"="dio") -> ("error out"=w348:errorcluster)  [unwired: 8 in]
              }
            }
            n200 = disable-structure shown="Enabled" {
              disable-tunnel: w328 -> [w344 _]
              disable-tunnel: w327 -> [w343 w345]
              disable-tunnel: [w342 w345] -> w326
              frame Disabled {
                n201 = Merge Errors(w344, w343) -> (w342:errorcluster)
              }
              frame Enabled {
              }
            }
          }
          frame 32 {
            # "update encoders"
            n202 = call <vilib>:"WPI_EncoderRefNum Registry Get.vi"("refnum name"="pickup arm") -> ("error out"=w391:errorcluster, "EncoderDevRef"=w390:T27)  [unwired: 9 in]
            n203 = call <vilib>:"WPI_EncoderRefNum Registry Get.vi"("refnum name"="right") -> ("error out"=w396:errorcluster, "EncoderDevRef"=w395:T27)  [unwired: 9 in]
            n204 = call <vilib>:"WPI_EncoderRefNum Registry Get.vi"("refnum name"="left") -> ("error out"=w393:errorcluster, "EncoderDevRef"=w394:T27)  [unwired: 9 in]
            n205 = call <vilib>:"WPI_EncoderGet.vi"("error in (no error)"=w396, "EncoderDevRef"=w395) -> ("Distance"=w388:dbl, "Rate"=w387:dbl)  [unwired: 4 in, 4 out]
            n206 = call <vilib>:"WPI_EncoderGet.vi"("error in (no error)"=w393, "EncoderDevRef"=w394) -> ("Distance"=w386:dbl, "Rate"=w385:dbl)  [unwired: 4 in, 4 out]
            n207 = call <vilib>:"WPI_EncoderGet.vi"("error in (no error)"=w391, "EncoderDevRef"=w390) -> ("Distance"=w384:dbl, "Rate"=w383:dbl)  [unwired: 4 in, 4 out]
            n208 = Build Array(w388, w387, w386, w385, w384, w383) -> (w382:dbl[])
            n209 = call <vilib>:"NT Write Numeric Array.vi"("Numeric Array"=w382, "Name"="encoders") -> ("error out"=w381:errorcluster)  [unwired: 9 in]
            n210 = disable-structure shown="Enabled" {
              disable-tunnel: w381 -> [w401 _]
              disable-tunnel: [w400 w402] -> w380
              disable-tunnel: w379 -> [w399 w402]
              frame Disabled {
                n211 = Merge Errors(w401, w399) -> (w400:errorcluster)
              }
              frame Enabled {
              }
            }
          }
          frame 37 {
            # "update motor array"
            n212 = call <vilib>:"WPI_MotorControlRefNum Registry Get.vi"("refnum name"="belts") -> ("error out"=w410:errorcluster, "MotorControlDevRef"=w412:T31)  [unwired: 9 in]
            n213 = call <vilib>:"WPI_MotorControlGetOutput.vi"("error in (no error)"=w410, "MotorControlDevRef"=w412) -> ("error out"=w405:errorcluster, "Output"=w409:dbl)  [unwired: 7 in, 1 out]
            n214 = call <vilib>:"NT Write Number.vi"("error in"=w405, "Numeric"=w409, "Name"="belts") -> ("error out"=w404:errorcluster)  [unwired: 8 in]
            n215 = disable-structure shown="Enabled" {
              disable-tunnel: [w415 w416] -> w407
              disable-tunnel: w406 -> [w414 w416]
              disable-tunnel: w404 -> [w413 _]
              frame Disabled {
                n216 = Merge Errors(w414, w413) -> (w415:errorcluster)
              }
              frame Enabled {
              }
            }
          }
          frame 40 {
            # "The solenoids are pretty fast, so all are read on call 40."
            n217 = Unbundle(w429) -> ("Solenoid Module"=w430:bool)  [unwired: 4 out]
            n218 = call <vilib>:"NT Read Number.vi"("Name"="solenoids") -> ("error out"=w419:errorcluster, "Numeric"=w426:dbl)  [unwired: 9 in]
            n219 = To Unsigned Byte Integer(number=w426) -> (unsigned 8bit integer=w424:u8)
            n220 = case shown="True" w430 {
              tunnel: [w436 w440] -> w428
              tunnel: w424 -> [w436 _]
              tunnel: [w435 w438] -> w420
              tunnel: w419 -> [w435 w437]
              frame False {
              }
              frame True {
                n221 = call <vilib>:"FPGA_SolenoidOpen.vi"("error in (no error)"=w437) -> ("error out"=w439:errorcluster, "SolenoidDevRef"=w441:T22)  [unwired: 1 in, 8 out]
                n222 = call <vilib>:"FPGA_SolenoidReadD07_0.vi"("error in (no error)"=w439, "SolenoidDevRef"=w441) -> ("error out"=w438:errorcluster, "DO7:0"=w440:u8)  [unwired: 8 out]
              }
            }
            n223 = To Double Precision Float(number=w428) -> (double precision float=w423:dbl)
            n224 = call <vilib>:"NT Write Number.vi"("error in"=w420, "Numeric"=w423, "Name"="solenoids") -> ("error out"=w421:errorcluster)  [unwired: 8 in]
            n225 = disable-structure shown="Enabled" {
              disable-tunnel: [w433 w434] -> w422
              disable-tunnel: w421 -> [w432 _]
              disable-tunnel: w418 -> [w431 w434]
              frame Disabled {
                n226 = Merge Errors(w432, w431) -> (w433:errorcluster)
              }
              frame Enabled {
              }
            }
          }
          frame 45 {
            w457 = fg_typedef."Get" ("Menu")
            n227 = call "dash safety data FG.vi"("Menu"=w457) -> ("Safety Data Out"=w443:T10)  [unwired: 1 in]
            n228 = call <vilib>:"RT Get CPU Loads.vi"() -> ("error out"=w447:errorcluster, "CPU loads"=w462:T37[])  [unwired: 10 in]
            n229 = call "performance fg.vi"("Menu"=w457) -> ("Output"=w461:T38)  [unwired: 1 in]
            n230 = call "vision data fg.vi"("Menu"=w457) -> ("Output"=w460:T15)  [unwired: 1 in]
            n231 = call "vision_fg.vi"("Menu"=w457) -> ("Enabled?"=w455:bool)  [unwired: 2 in, 1 out]
            n232 = Unbundle(w460) -> ("Hot Goal Present?"=w459:bool, "distance"=w458:dbl)  [unwired: 5 out]
            n233 = Index Array(array=w462) -> (element=w463:T37)  [unwired: 1 in]
            n234 = Unbundle By Name(w463) -> ("Total (%)"=w451:dbl)
            n235 = Unbundle By Name(w461) -> ("Vision mSPI"=w452:u32, "Main mSPI"=w453:u32)
            n236 = Bundle("Hot Goal Present?"=w459, "distance"=w458) -> (w454:T26)  [unwired: 1 in]
            n237 = Bundle By Name(cluster=T9 {"Total (%)"=0.0, "Vision mSPI"=0, "Main mSPI"=0, "Vision"={"Hot Goal Present?"=FALSE, "distance"=0.0}, "Enabled?"=FALSE, "Safety Data"={"At Distance Limit"=FALSE, "No Rate Read"=FALSE, "Encoder Disconnected"=FALSE, "Encoder Directional Issue"=FALSE}}, "Safety Data"=w443, "Total (%)"=w451, "Vision mSPI"=w452, "Main mSPI"=w453, "Vision"=w454, "Enabled?"=w455) -> (w442:T9)
            n238 = Flatten To String(anything=w442, error in (no error)=w447) -> (data string=w450:string, error out=w448:errorcluster)  [unwired: 3 out]
            n239 = call <vilib>:"NT Write String.vi"("error in"=w448, "String"=w450, "Name"="dashdata") -> ("error out"=w446:errorcluster)  [unwired: 8 in]
            n240 = disable-structure shown="Enabled" {
              disable-tunnel: w446 -> [w466 _]
              disable-tunnel: [w465 w467] -> w445
              disable-tunnel: w444 -> [w464 w467]
              frame Disabled {
                n241 = Merge Errors(w466, w464) -> (w465:errorcluster)
              }
              frame Enabled {
              }
            }
          }
          frame 47 {
            n242 = call "timeout error fg.vi"() -> ("# of Timeouts"=w481:u32, "Time Out Error This Match"=w480:bool)  [unwired: 2 in]
            n243 = call "safe shoot error.vi"("Menu"=fg_typedef."Get") -> ("Can Shoot Safely?"=w477:bool)  [unwired: 1 in]
            n244 = Bundle By Name(cluster=T6 {"# of Timeouts"=0, "Time Out Error This Match"=FALSE}, "Time Out Error This Match"=w480, "# of Timeouts"=w481) -> (w478:T6)
            n245 = Bundle By Name(cluster=T11 {"Timeout Data"={"# of Timeouts"=0, "Time Out Error This Match"=FALSE}, "Can Shoot Safely?"=FALSE}, "Timeout Data"=w478, "Can Shoot Safely?"=w477) -> (w476:T11)
            n246 = Flatten To String(anything=w476) -> (data string=w472:string, error out=w474:errorcluster)  [unwired: 1 in, 3 out]
            n247 = call <vilib>:"NT Write String.vi"("error in"=w474, "String"=w472, "Name"="errors") -> ("error out"=w470:errorcluster)  [unwired: 8 in]
            n248 = disable-structure shown="Enabled" {
              disable-tunnel: [w485 w486] -> w471
              disable-tunnel: w470 -> [w484 _]
              disable-tunnel: w469 -> [w483 w486]
              frame Disabled {
                n249 = Merge Errors(w484, w483) -> (w485:errorcluster)
              }
              frame Enabled {
              }
            }
          }
        }
      }
      "Errors" <- w240
    }
  }
